vi "search for tag.vi"(8 "error in":errorcluster, 10 "system tag":refnum<class "data bus tag description.lvclass">, 11 "data dictionary in":refnum<class "data bus dictionary.lvclass">) -> (0 "error out":errorcluster, 2 "index":i32, 3 "data dictionary out":refnum<class "data bus dictionary.lvclass">)   [LabVIEW 2013, in "data bus dictionary.lvclass"]
doc: "Uses a tag descriptor to locate a tag within the dictionary. This function uses the name and data type fields of the descriptor."
uses:
  data bus dictionary.lvclass
  tag/data bus tag description.lvclass
  tag/data bus tag description.lvclass/data bus tag description.ctl
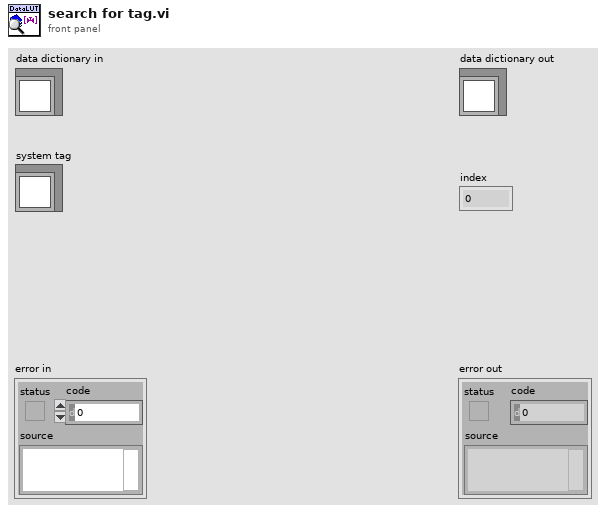
[diagram p1: front panel]
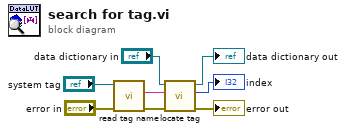
[diagram p0: block diagram]
diagram:
  n1 = call "read tag name.vi"("error in"="error in", "system tag in"="system tag") -> ("error out"=w6:errorcluster, "name"=w3:string)  [unwired: 7 in, 1 out]
  n2 = call "locate tag.vi"("error in"=w6, "name"=w3, "data dictionary in"="data dictionary in") -> ("error out"=→"error out":errorcluster, "index"=→"index":i32, "data dictionary out"=→"data dictionary out":refnum<class "data bus dictionary.lvclass">)  [unwired: 5 in, 1 out]
